vi "SETPINSTATUS.vi"(0 "Serial Device in":refnum<class "Serial Device.lvclass">, 5 "PORT":dbl, 7 "PIN":dbl, 9 "valor":bool, 11 "error in (no error)":errorcluster) -> (4 "Serial Device out":refnum<class "Serial Device.lvclass">, 15 "error out":errorcluster)   [LabVIEW 2019, in "Serial Device.lvclass"]
uses:
  Serial Device.lvclass
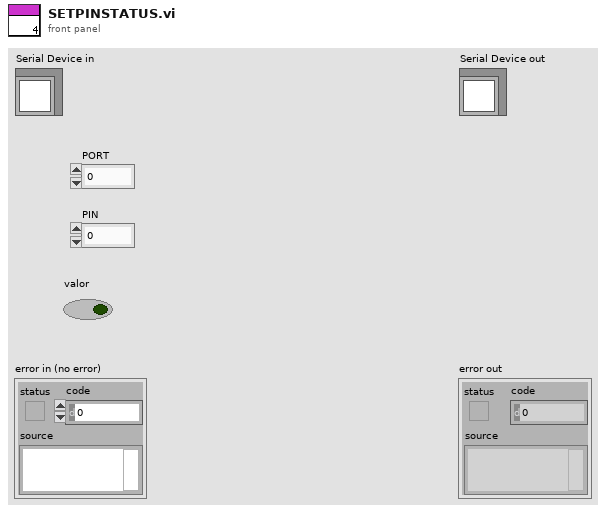
[diagram p1: front panel]
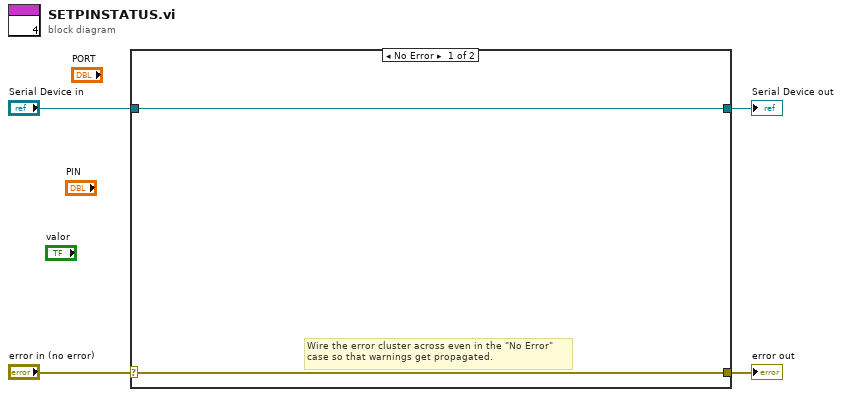
[diagram p0: block diagram]
diagram:
  n1 = case shown="No Error" "error in (no error)" {
    selector: "error in (no error)" -> [w5 w8]
    tunnel: [w5 w8] -> w3
    tunnel: [w6 w7] -> w1
    tunnel: "Serial Device in" -> [w6 w7]
    frame No Error {
      # "Wire the error cluster across even in the \"No Error\"\ncase so that warnings get propagated."
    }
    frame Error {
    }
  }
  "error out" <- w3
  "Serial Device out" <- w1
